vi "MS Elapsed.vi"(11 "ms in":u32) -> (2 "elapsed ms":u32, 3 "new ms time":u32)   [LabVIEW 2013]
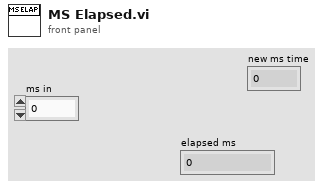
[diagram p1: front panel]
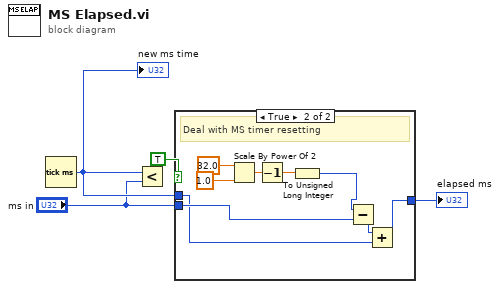
[diagram p0: block diagram]
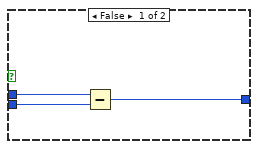
[diagram p2: hidden frame]
diagram:
  n1 = Tick Count (ms)() -> (millisecond timer value=w3:u32)
  "new ms time" <- w3
  n2 = Less?(x=w3, y="ms in") -> ()  [unwired: 1 out]
  n3 = case shown="True" TRUE {
    tunnel: [w7 w11] -> w4
    tunnel: w3 -> [w6 w12]
    tunnel: "ms in" -> [w5 w14]
    frame False {
      n4 = Subtract(x=w6, y=w5) -> (x-y=w7:u32)
    }
    frame True {
      # "Deal with MS timer resetting"
      n5 = Scale By Power Of 2(n=32.0, x=1.0 ("millisecond timer value in")) -> (x*2^n=w10:dbl)
      n6 = Decrement(x=w10) -> (x-1=w9:dbl)
      n7 = To Unsigned Long Integer(number=w9) -> (unsigned 32bit integer=w8:u32)
      n8 = Subtract(x=w8, y=w14) -> (x-y=w13:u32)
      n9 = Add(x=w13, y=w12) -> (x+y=w11:u32)
    }
  }
  "elapsed ms" <- w4
